vi "SRV_PM_Data Field Length.vi"(0 "Data":u8[](array[numeric]), 11 "error in (no error)":errorcluster, 12 "Data Field Length Number of Bytes (2)":i32=2, 13 "Generate Error if Data Too Long (T)":bool=TRUE) -> (4 "Data dup":u8[](array[numeric]), 8 "Data Field Length Bytes":u8[](array[numeric]), 15 "error out":errorcluster)   [LabVIEW 2014]
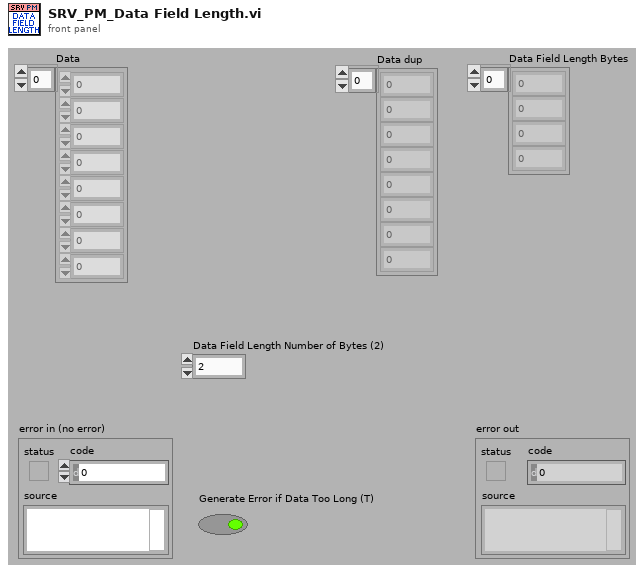
[diagram p1: front panel]
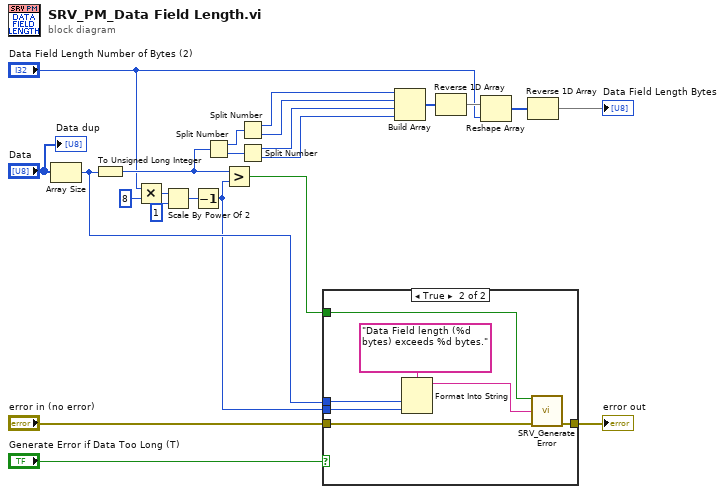
[diagram p0: block diagram]
diagram:
  n1 = Array Size(array="Data") -> (size(s)=w3:i32)
  n2 = To Unsigned Long Integer(number=w3) -> (unsigned 32bit integer=w22:u32)
  n3 = Multiply(x="Data Field Length Number of Bytes (2)", y=8 ("x")) -> (x*y=w11:i32)
  n4 = Scale By Power Of 2(n=w11, x=u32 1) -> (x*2^n=w10:u32)
  n5 = Decrement(x=w10) -> (x-1=w2:u32)
  n6 = Split Number(x=w22) -> (hi(x)=w21:u16, lo(x)=w23:u16)
  n7 = Greater?(x=w22, y=w2) -> (0:w7:bool)
  n8 = Split Number(x=w21) -> (hi(x)=w20:u8, lo(x)=w19:u8)
  n9 = Split Number(x=w23) -> (hi(x)=w18:u8, lo(x)=w17:u8)
  n10 = case shown="True" "Generate Error if Data Too Long (T)" {
    tunnel: w7 -> [_ w29]
    tunnel: "error in (no error)" -> [w24 w28]
    tunnel: [w24 w27] -> w5
    tunnel: w3 -> [_ w26]
    tunnel: w2 -> [_ w25]
    frame False {
    }
    frame True {
      n11 = Format Into String(format string="Data Field length (%d bytes) exceeds %d bytes." ("Message"), w26, w25) -> (resulting string=w30:string)  [unwired: 2 in, 1 out]
      n12 = call "SRV_Generate Error.vi"("status (T)"=w29, "Message"=w30, "error in (no error)"=w28) -> ("error out"=w27:errorcluster)  [unwired: 12 in]
    }
  }
  "error out" <- w5
  n13 = Build Array(w20, w19, w18, w17) -> (w16:u8[])
  n14 = Reverse 1D Array(array=w16) -> (reversed array=w15:u8[])
  n15 = Reshape Array(w15, "Data Field Length Number of Bytes (2)") -> (w14:u8[])
  n16 = Reverse 1D Array(array=w14) -> (reversed array=→"Data Field Length Bytes":u8[])
  "Data dup" <- "Data"
